vi "setCornerWidget.vi"(8 "Error In":errorcluster, 9 "corner":T1 items=["TopLeftCorner", "TopRightCorner", "BottomLeftCorner", "BottomRightCorner"], 10 "widget":refnum<class "QWidget.lvclass">, 11 "QTabWidget In":refnum<class "QTabWidget.lvclass">) -> (0 "Error Out":errorcluster, 3 "QTabWidget Out":refnum<class "QTabWidget.lvclass">)   [LabVIEW 2014, in "QTabWidget.lvclass"]
doc: "LabVIEW-specific documentation is not yet available. See <b>http://doc.qt.io/qt-5/QTabWidget.html#setCornerWidget</b>"
uses:
  QTabWidget.lvclass
  QWidget/QWidget.lvclass
  LQ Core/Qt/Corner.ctl
  LQ Core/LQIdentity/LQIdentity.lvclass/LQIdentity.ctl
  LQ Core/LQ Core.lvlib
  LQ Core/LQIdentity/LQIdentity.lvclass
  LQ Core/Qt/Qt.lvlib
panel:
  # "Copyright (c) 2016 Sze Howe Koh\n\nThis Source Code Form is subject to the terms of the Mozilla Public\nLicense, v. 2.0. If a copy of the MPL was not distributed with this\nfile, You can obtain one at http://mozilla.org/MPL/2.0/."
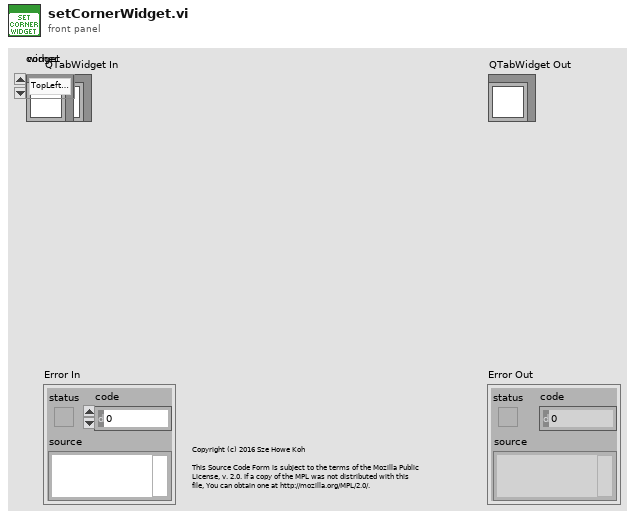
[diagram p1: front panel]
types:
  T1 = typedef "Qt.lvlib/Corner.ctl" = i32
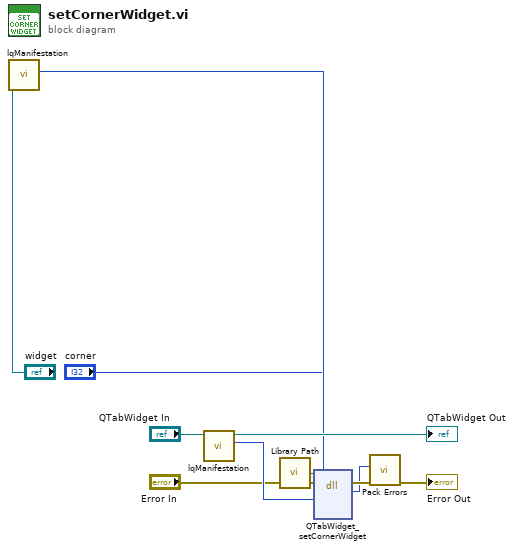
[diagram p0: block diagram]
diagram:
  n1 = call "lqManifestation.vi"("LQIdentity in"="widget") -> ("Manifestation"=w2:u64)  [unwired: 9 in, 1 out]
  n2 = call "lqManifestation.vi"("LQIdentity in"="QTabWidget In") -> ("Manifestation"=w8:u64, "LQIdentity out"=→"QTabWidget Out":refnum<class "QTabWidget.lvclass">)  [unwired: 9 in]
  n3 = call "Library Path.vi"() -> ("Library Path"=w9:path)
  n4 = dll-call lib="?" fn="QTabWidget_setCornerWidget"(path in=w9, error in="Error In", "_instance"=w8, "widget"=w2, "corner"="corner") -> (error out=w6:errorcluster, w4:i32)  [unwired: 4 in, 1 out]
  n5 = call "Pack Errors.vi"("Error In"=w6, "Error Code"=w4) -> ("Error Out"=→"Error Out":errorcluster)  [unwired: 9 in]
